vi "Tektronix DPO MSO 2000 4000 Series Acquire Waveform Example.vi"() -> ()   [LabVIEW 2016]
doc: "This example illustrates how to use autosetup and acquire a waveform on a single channel using the following steps:\n\n1. Specify a valid VISA session. \n2. Specify a channel. \n3. Specify a time-out value for reading waveform.\n4. Run the VI. The graph displays the waveform you acquire."
uses:
  <instrlib>/Tektronix DPO MSO 2000 4000 Series/Public/Data/Read (Single Waveform).vi
  <instrlib>/Tektronix DPO MSO 2000 4000 Series/Tektronix DPO MSO 2000 4000 Series.lvlib
panel:
  in  "Channel (0: Channel 1)":u16(ring) items=["Channel 1", "Channel 2", "Channel 3", "Channel 4", "Math", "Reference 1", "Reference 2", "Reference 3", "Reference 4", "D0", "D1", "D2", "D3", "D4", "D5", "D6", "D7", "D8", "D9", "D10", "D11", "D12", "D13", "D14", "D15", "Amplitude", "Frequency", "Phase", "Normal", "Average", "Maximum Peak Hold", "Minimum Peak Hold"]
  in  "Maximum Time (10000ms)":u32=10000
  in  "VISA Resource Name":refnum<visa-resource-name>
  out "Waveform Graph":waveform(dbl)(graph)
  # "(C) 2006 - 2016. National Instruments Corporation. ALL RIGHTS RESERVED."
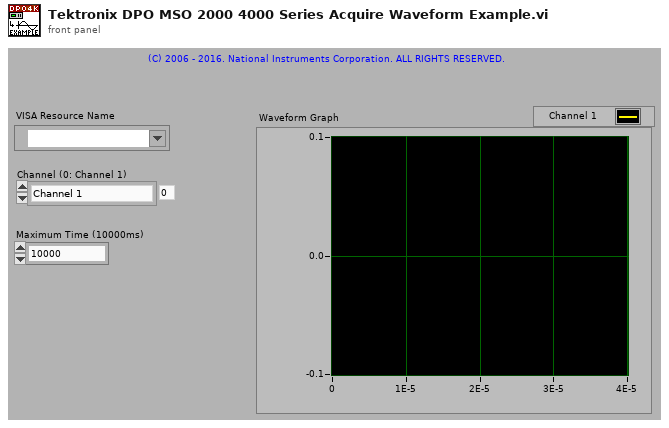
[diagram p1: front panel]
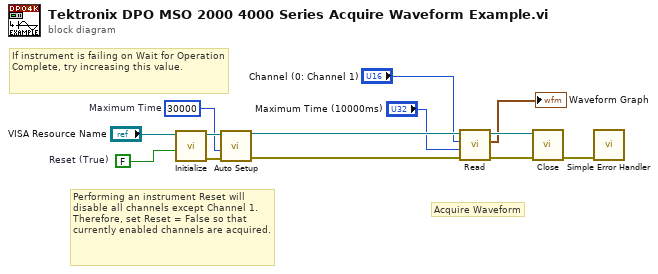
[diagram p0: block diagram]
diagram:
  w2 = u32 30000  # Maximum Time
  w6 = FALSE  # Reset (True)
  # "If instrument is failing on Wait for Operation Complete, try increasing this value."
  # "Performing an instrument Reset will disable all channels except Channel 1. Therefore, set Reset = False so that currently enabled channels are acquired."
  # "Acquire Waveform"
  n1 = call <instrlib>:"Initialize.vi"("Reset (True)"=w6, "VISA resource name"="VISA Resource Name") -> ("error out"=w7:errorcluster, "VISA resource name out"=w8:refnum<visa-resource-name>)  [unwired: 8 in]
  n2 = call <instrlib>:"Auto Setup.vi"("error in (no error)"=w7, "Maximum Time (10000ms)"=w2, "VISA resource name"=w8) -> ("error out"=w3:errorcluster, "VISA resource name out"=w5:refnum<visa-resource-name>)  [unwired: 7 in]
  n3 = call-poly <instrlib>:"Read.vi"("error in (no error)"=w3, "Maximum Time (10000ms)"="Maximum Time (10000ms)", "Channel (0: Channel 1)"="Channel (0: Channel 1)", "VISA resource name"=w5) -> ("error out"=w10:errorcluster, "Waveform Graph"=→"Waveform Graph":waveform(dbl), "VISA resource name out"=w11:refnum<visa-resource-name>)  [unwired: 5 in]
  n4 = call <instrlib>:"Close.vi"("error in (no error)"=w10, "VISA resource name"=w11) -> ("error out"=w12:errorcluster)  [unwired: 9 in]
  n5 = call <vilib>:"Simple Error Handler.vi"("error in (no error)"=w12) -> ()  [unwired: 4 in, 5 out]
